vi "Set VDI sweep parameters.vi"(5 "MW generator constants":T2[](array[typedef]), 9 "Sweep parameters":T3 {"Sweep down\ntime [ms]" min=0.0 max=250.0; "End [GHz]" min=8.0 max=20.0; "Intermidiate [MHz]" min=0.0 max=2500.0; "Start [GHz]" min=8.0 max=20.0}) -> (4 "data out1":u8[][](array[numeric]), 6 "data out 2":u8[][](array[numeric]), 8 "Freq limit reached":bool, 10 "Error1":bool, 15 "Error2":bool)   [LabVIEW 2022 SP3, in "THz source modeule.lvlib"]
uses:
  THz source modeule.lvlib
  ctl/THz sweep parameters.ctl
  ctl/THz MW generator constants.ctl
panel:
  out "Folower Actual settings":T1 {"CWFreq(GHz)" format="%#_12g"; "RiseStepDwellTime(uS)" format="%#_12g"; "FallStepDwellTime(uS)" format="%#_12g"; "RiseTime(mS)" format="%#_14g"; "FallTime(mS)" format="%#_14g"; "StartFreq(GHz)" format="%#_12g"; "StopFreq(GHz)" format="%#_12g"; "RiseStepSize(Hz)" format="%#_12g"; "FallStepSize(Hz)" format="%#_12g"; "Rise#Steps" format="%#_12g"; "Fall#Steps" format="%#_12g"}
  out "Actual settings":T1 {"CWFreq(GHz)" format="%#_12g"; "RiseStepDwellTime(uS)" format="%#_12g"; "FallStepDwellTime(uS)" format="%#_12g"; "RiseTime(mS)" format="%#_14g"; "FallTime(mS)" format="%#_14g"; "StartFreq(GHz)" format="%#_12g"; "StopFreq(GHz)" format="%#_12g"; "RiseStepSize(Hz)" format="%#_12g"; "FallStepSize(Hz)" format="%#_12g"; "Rise#Steps" format="%#_12g"; "Fall#Steps" format="%#_12g"}
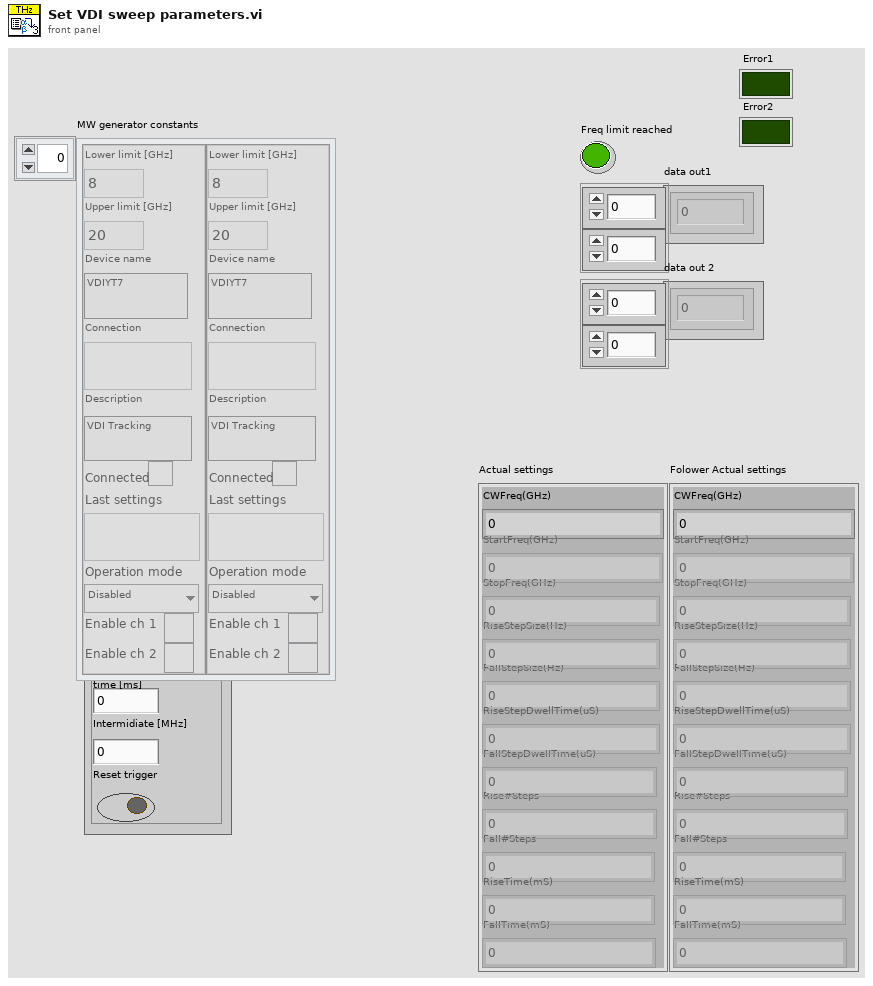
[diagram p1: front panel]
types:
  T1 = cluster{"CWFreq(GHz)":dbl, "StartFreq(GHz)":dbl, "StopFreq(GHz)":dbl, "RiseStepSize(Hz)":dbl, "FallStepSize(Hz)":dbl, "RiseStepDwellTime(uS)":dbl, "FallStepDwellTime(uS)":dbl, "Rise#Steps":dbl, "Fall#Steps":dbl, "RiseTime(mS)":dbl, "FallTime(mS)":dbl}
  T2 = typedef "THz source modeule.lvlib/THz MW generator constants.ctl" = cluster{"Lower limit [GHz]":dbl, "Upper limit [GHz]":dbl, "Device name":string, "Connection":string, "Description":string, "Connected":bool, "Last settings":string, "Operation mode":enum16{"Disabled", "CW", "Arbitrary", "Sweep"}, "Enable ch 1":bool, "Enable ch 2":bool}
  T3 = typedef "THz source modeule.lvlib/THz sweep parameters.ctl" = cluster{"Start [GHz]":dbl, "End [GHz] ":dbl, "Sweep up\ntime [ms]":dbl, "Sweep down\ntime [ms]":dbl, "Intermidiate [MHz]":dbl, "Reset trigger":bool}
  T4 = cluster{"Numeric Control":dbl, "Numeric Control":dbl, i32, i32, i32, i32, "RiseFall Dwell Low":bool, "RiseFall Dwell High":bool, "Pause Sweep":bool, "Swep Direction":bool}
  T5 = cluster{"Lowest Sweep Frequency(GHz)":dbl, "Highest Sweep Frequency(GHz)":dbl, "Rising Step Size(GHz)":dbl, "Falling Step Size(GHz)":dbl, "Rising Step Time(uS)":dbl, "Falling Step Time(uS)":dbl, "Dwell Low":bool, "Dwell High":bool, "Sweep Pause":bool, "Sweep Direction":bool}
  T6 = cluster{"Upper limit [GHz]":dbl, "Upper limit [GHz]":dbl, i32, i32, i32, i32, bool, bool, bool, bool}
  T7 = cluster{"Upper limit [GHz]":dbl, "Upper limit [GHz]":dbl, i32, i32, i32, i32, bool, bool, bool, bool}[]
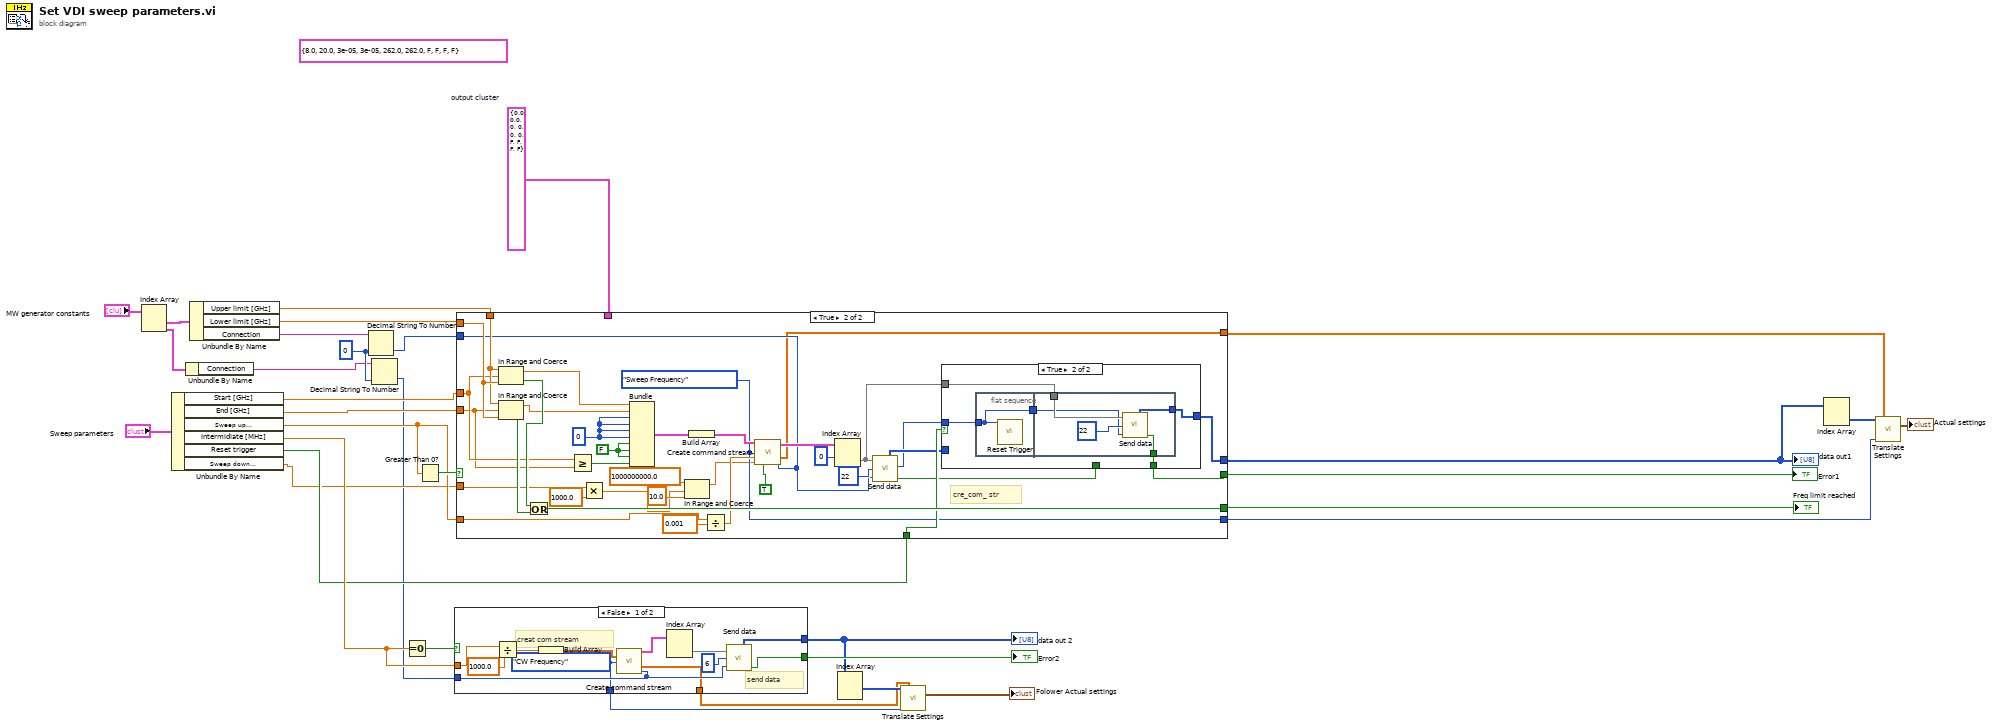
[diagram p0: block diagram]
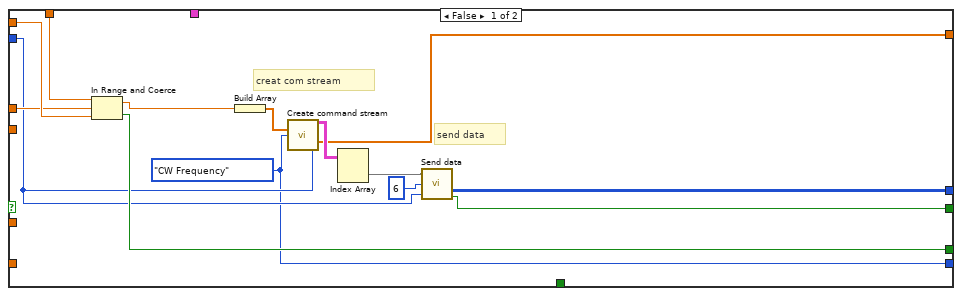
[diagram p3: hidden frame]
diagram:
  w3 = u64 0 ("default (0 I32)")
  w21 = T4 {"Numeric Control"=0.0, "Numeric Control"=0.0, 0, 0, 0, 0, "RiseFall Dwell Low"=FALSE, "RiseFall Dwell High"=FALSE, "Pause Sweep"=FALSE, "Swep Direction"=FALSE}  # output cluster
  (unwired) T5 {"Lowest Sweep Frequency(GHz)"=8.0, "Highest Sweep Frequency(GHz)"=20.0, "Rising Step Size(GHz)"=3e-05, "Falling Step Size(GHz)"=3e-05, "Rising Step Time(uS)"=262.0, "Falling Step Time(uS)"=262.0, "Dwell Low"=FALSE, "Dwell High"=FALSE, "Sweep Pause"=FALSE, "Sweep Direction"=FALSE} ("Sweep Parameters")
  n1 = Index Array(array="MW generator constants") -> (element #1=w6:T2, element #2=w4:T2)  [unwired: 2 in]
  n2 = Unbundle By Name("Sweep parameters") -> ("Start [GHz]"=w25:dbl, "End [GHz]"=w27:dbl, "Sweep up\ntime [ms]"=w23:dbl, "Intermidiate [MHz]"=w32:dbl, "Reset trigger"=w20:bool, "Sweep down\ntime [ms]"=w13:dbl)
  n3 = Unbundle By Name(w4) -> ("Connection"=w2:string)
  n4 = Unbundle By Name(w6) -> ("Upper limit [GHz]"=w28:dbl, "Lower limit [GHz]"=w26:dbl, "Connection"=w19:string)
  n5 = Decimal String To Number(string=w19, default (0L)=w3) -> (number=w5:u64)  [unwired: 1 in, 1 out]
  n6 = Decimal String To Number(string=w2, default (0L)=w3) -> (number=w1:u64)  [unwired: 1 in, 1 out]
  n7 = Equal To 0?(x=w32) -> (x = 0?=w31:bool)
  n8 = Greater Than 0?(x=w23) -> (x > 0?=w24:bool)
  n9 = case shown="False" w31 {
    tunnel: w1 -> [w40 _]
    tunnel: w32 -> [w45 _]
    tunnel: [w39 _] -> w33
    tunnel: [w38 _] -> w12
    tunnel: [w35 _] -> w10
    tunnel: [w34 _] -> w9
    frame False {
      w34 = enum16{"CW Frequency", "Sweep Frequency"}."CW Frequency" ("Command mode")
      # "send data"
      # "creat com stream"
      n10 = Divide(x=w45, y=1000.0) -> (x/y=w37:dbl)
      n11 = Build Array(w37) -> (w43:dbl[])
      n12 = call <instrlib>:"Create command stream.vi"("CWfreq array(GHz)"=w43, "Command mode"=w34, "Handle"=w40) -> ("Data packets"=w44:cluster{"Write Data":u8[]}[][], "Output step time(uS)"=w35:dbl[])  [unwired: 11 in]
      n13 = Index Array(array=w44) -> (element=w42:cluster{"Write Data":u8[]}[])  [unwired: 2 in]
      n14 = call <instrlib>:"Send data.vi"("Data packets"=w42, "bytes to read"=6 ("index"), "Handle"=w40) -> ("data out"=w38:u8[][], "Error"=w39:bool)  [unwired: 3 in, 3 out]
    }
    frame True {
      # "No following synth"
    }
  }
  "Error2" <- w33
  "data out 2" <- w12
  n15 = case shown="True" w24 {
    tunnel: w25 -> [w57 w78]
    tunnel: w26 -> [w58 w96]
    tunnel: w27 -> [_ w77]
    tunnel: w28 -> [w59 w95]
    tunnel: w21 -> [_ _]
    tunnel: w23 -> [_ w75]
    tunnel: w5 -> [w49 w74]
    tunnel: [w50 w70] -> w29
    tunnel: [w55 w86] -> w22
    tunnel: [w51 w69] -> w18
    tunnel: w20 -> [_ w79]
    tunnel: [w47 w67] -> w16
    tunnel: [w46 w66] -> w15
    tunnel: w13 -> [_ w64]
    frame False {
      w46 = enum16{"CW Frequency", "Sweep Frequency"}."CW Frequency" ("Command mode")
      # "send data"
      # "creat com stream"
      n16 = In Range and Coerce(upper limit=w59, x=w57, lower limit=w58) -> (coerced(x)=w56:dbl, In Range?=w55:bool)
      n17 = Build Array(w56) -> (w48:dbl[])
      n18 = call <instrlib>:"Create command stream.vi"("CWfreq array(GHz)"=w48, "Command mode"=w46, "Handle"=w49) -> ("Data packets"=w54:cluster{"Write Data":u8[]}[][], "Output step time(uS)"=w47:dbl[])  [unwired: 11 in]
      n19 = Index Array(array=w54) -> (element=w53:cluster{"Write Data":u8[]}[])  [unwired: 2 in]
      n20 = call <instrlib>:"Send data.vi"("Data packets"=w53, "bytes to read"=6 ("index"), "Handle"=w49) -> ("data out"=w51:u8[][], "Error"=w50:bool)  [unwired: 3 in, 3 out]
    }
    frame True {
      w66 = enum16{"CW Frequency", "Sweep Frequency"}."Sweep Frequency" ("Command mode")
      w91 = FALSE
      w92 = 0
      # "cre_com_ str"
      n21 = In Range and Coerce(upper limit=w95, x=w78, lower limit=w96) -> (coerced(x)=w89:dbl, In Range?=w94:bool)
      n22 = In Range and Coerce(upper limit=w95, x=w77, lower limit=w96) -> (coerced(x)=w88:dbl, In Range?=w93:bool)
      n23 = Or(x=w94, y=w93) -> (x .or. y?=w86:bool)
      n24 = Greater Or Equal?(x=w78, y=w77) -> (x >= y?=w76:bool)
      n25 = Multiply(x=w64, y=1000.0 ("Sweep down\ntime [ms]")) -> (x*y=w61:dbl)
      n26 = Bundle("Upper limit [GHz]"=w89, "Upper limit [GHz]"=w88, w92, w92, w92, w92, w91, w91, w91, w76) -> (w90:T6)  [unwired: 1 in]
      n27 = In Range and Coerce(upper limit=1000000000.0, x=w61, lower limit=10.0) -> (coerced(x)=w65:dbl)  [unwired: 1 out]
      n28 = Build Array(w90) -> (w85:T7)
      n29 = Divide(x=w75, y=0.001) -> (x/y=w83:dbl)
      n30 = call <instrlib>:"Create command stream.vi"("Sweep Parameters"=w85, "Command mode"=w66, "Rising Sweep Time(uS)"=w83, "Falling Sweep Time(uS)"=w65, "Calculate step size,time"=TRUE, "Handle"=w74) -> ("Data packets"=w84:cluster{"Write Data":u8[]}[][], "Output step time(uS)"=w67:dbl[])  [unwired: 8 in]
      n31 = Index Array(array=w84, index (row)=0) -> (element=w72:cluster{"Write Data":u8[]}[])  [unwired: 1 in]
      n32 = call <instrlib>:"Send data.vi"("Data packets"=w72, "bytes to read"=u32 22, "Handle"=w74) -> ("data out"=w73:u8[][], "Handle out"=w71:u64, "Error"=w68:bool)  [unwired: 3 in, 2 out]
      n33 = case shown="True" w79 {
        tunnel: w71 -> [_ w103]
        tunnel: w73 -> [w98 _]
        tunnel: w72 -> [_ w102]
        tunnel: [w97 w101] -> w70
        tunnel: [w98 w100] -> w69
        tunnel: w68 -> [w97 _]
        frame False {
        }
        frame True {
          n34 = flat-sequence {
            tunnel: w103 -> [w104]
            tunnel: [w104] -> w99
            tunnel: w102 -> [w109]
            tunnel: [w107] -> w101
            tunnel: [w106] -> w100
            tunnel: w99 -> [w105]
            frame #0 {
              n35 = call <instrlib>:"Reset Trigger.vi"("Handle"=w104) -> ()  [unwired: 11 in]
            }
            frame #1 {
              n36 = call <instrlib>:"Send data.vi"("Data packets"=w109, "bytes to read"=u32 22, "Handle"=w105) -> ("data out"=w106:u8[][], "Error"=w107:bool)  [unwired: 3 in, 3 out]
            }
          }
        }
      }
    }
  }
  "Error1" <- w29
  "Freq limit reached" <- w22
  "data out1" <- w18
  n37 = Index Array(array=w12) -> (element=w11:u8[])  [unwired: 2 in]
  n38 = call "Translate Settings.vi"("data"=w11, "Step time(uS)"=w10, "Command mode"=w9) -> ("Actual settings"=→"Folower Actual settings":T1)  [unwired: 12 in]
  n39 = Index Array(array=w18) -> (element=w17:u8[])  [unwired: 2 in]
  n40 = call "Translate Settings.vi"("data"=w17, "Step time(uS)"=w16, "Command mode"=w15) -> ("Actual settings"=→"Actual settings":T1)  [unwired: 12 in]
